vi "S2C_XML_UpdateMeasMeta.vi"(8 "Error In":errorcluster) -> (0 "Error Out":errorcluster)   [LabVIEW 2015]
uses:
  S2C_XML_Globals.vi
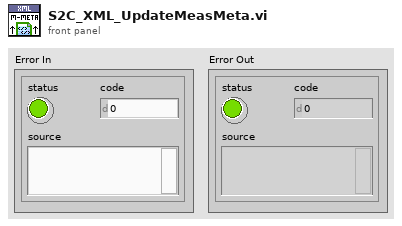
[diagram p1: front panel]
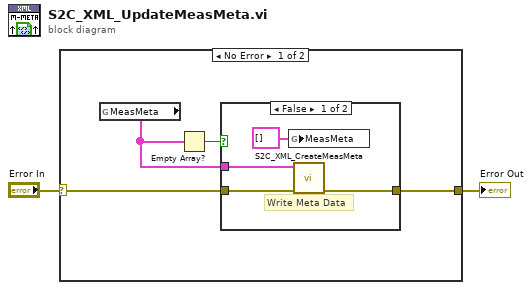
[diagram p0: block diagram]
diagram:
  n1 = case shown="No Error" "Error In" {
    selector: "Error In" -> [w6 w12]
    tunnel: [w5 w12] -> w2
    frame No Error {
      n2 = global read "S2C_XML_Globals.vi" "MeasMeta"() -> (w4:cluster{"MetaName":string, "MetaValue":string}[])
      n3 = Empty Array?(array=w4) -> (empty?=w3:bool)
      n4 = case shown="False" w3 {
        tunnel: w6 -> [w10 w11]
        tunnel: [w9 w11] -> w5
        tunnel: w4 -> [w8 _]
        frame False {
          # "Write Meta Data"
          n5 = global write "S2C_XML_Globals.vi" "MeasMeta"(cluster{"MetaName":string, "MetaValue":string}[] [] ("MeasMeta")) -> ()
          n6 = call "S2C_XML_CreateMeasMeta.vi"("Error In"=w10, "MetaArray"=w8) -> ("Error Out"=w9:errorcluster)  [unwired: 9 in]
        }
        frame True {
        }
      }
    }
    frame Error {
    }
  }
  "Error Out" <- w2
